vi "_PC_Daemon_Pref_SetExperimentCode.vi"(2 "error in (no error)":errorcluster, 3 "FileData":string) -> (0 "error out":errorcluster)   [LabVIEW 2018]
uses:
  RecipeEditor/Ctl/WfmCmd_Type.ctl
  PublicSubVI/Class/SigInfo/SigInfo.ctl
  PublicSubVI/Class/SigInfo/SigInfo.lvclass
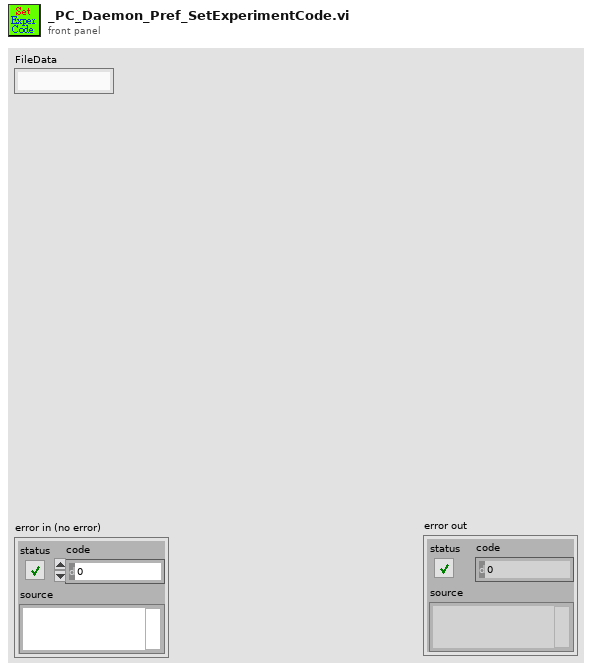
[diagram p1: front panel]
types:
  T1 = cluster{"ProcessCodes":u64[], "WfmCodes":u64[], "Signal Remarks":cluster{"mzID":u64, "SignalInfo":cluster{"Label":string, "dt":dbl, "Length":u32, "RefVolt":dbl, "mzTable":cluster{"t":dbl[], "mz":dbl[], "beta":dbl[]}}[]}, "scriptCode":string}
  T2 = typedef "SigInfo.ctl" = enum16{"New mzList", "Set SigInfo", "Get SigInfo", "Append", "End"}
  T3 = typedef "WfmCmd_Type.ctl" = enum8{"None", "WFM", "EventCodes"}
  T4 = cluster{"mzID":u64, "SignalInfo":cluster{"Label":string, "dt":dbl, "Length":u32, "RefVolt":dbl, "mzTable":cluster{"t":dbl[], "mz":dbl[], "beta":dbl[]}}[]}
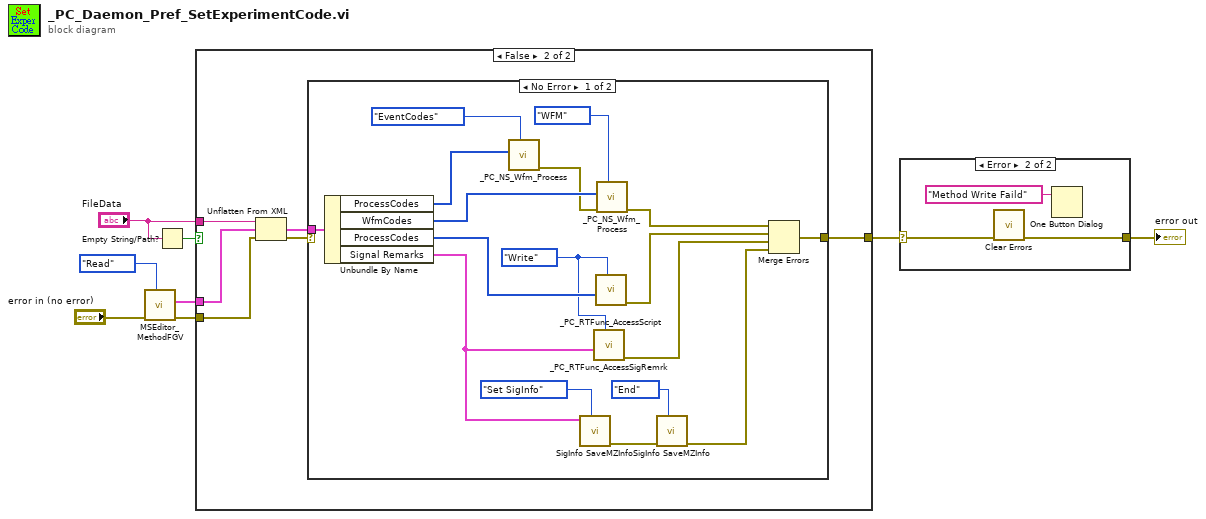
[diagram p0: block diagram]
diagram:
  n1 = call "MSEditor_MethodFGV.vi"("error in (no error)"="error in (no error)", "Function"=enum16{"Write", "Read"}."Read") -> ("Mthd out"=w4:T1, "error out"=w1:errorcluster)  [unwired: 7 in]
  n2 = Empty String/Path?(string/path="FileData") -> (empty?=w8:bool)
  n3 = case shown="False" w8 {
    tunnel: "FileData" -> [_ w14]
    tunnel: [_ w11] -> w6
    tunnel: w4 -> [_ w10]
    tunnel: w1 -> [_ w9]
    frame True {
    }
    frame False {
      n4 = Unflatten From XML(xml string=w14, type=w10, error in (no error)=w9) -> (value=w13:T1, error out=w12:errorcluster)
      n5 = case shown="No Error" w12 {
        selector: w12 -> [_ w32]
        tunnel: w13 -> [w27 _]
        tunnel: [w25 w32] -> w11
        frame No Error {
          w20 = enum16{"Write", "Read"}."Write" ("Function")
          n6 = Unbundle By Name(w27) -> ("ProcessCodes"=w29:u64[], "WfmCodes"=w28:u64[], "ProcessCodes"=w21:u64[], "Signal Remarks"=w19:T4)
          n7 = call "_PC_NS_Wfm_Process.vi"("Wfm_Type"=WfmCmd_Type."EventCodes", "WfmData_U64 in"=w29) -> ("error out"=w24:errorcluster)  [unwired: 9 in]
          n8 = call "SigInfo SaveMZInfo.vi"("Function"=SigInfo."Set SigInfo", "Signal Remarks input"=w19) -> ("error out"=w18:errorcluster)  [unwired: 7 in, 2 out]
          n9 = call "_PC_RTFunc_AccessSigRemrk.vi"("Function"=w20, "Var in"=w19) -> ("error out"=w22:errorcluster)  [unwired: 8 in, 1 out]
          n10 = call "_PC_RTFunc_AccessScript.vi"("Function"=w20, "Var in"=w21) -> ("error out"=w23:errorcluster)  [unwired: 8 in, 1 out]
          n11 = call "_PC_NS_Wfm_Process.vi"("Wfm_Type"=WfmCmd_Type."WFM", "error in (no error)"=w24, "WfmData_U64 in"=w28) -> ("error out"=w26:errorcluster)  [unwired: 8 in]
          n12 = call "SigInfo SaveMZInfo.vi"("Function"=SigInfo."End", "error in (no error)"=w18) -> ("error out"=w17:errorcluster)  [unwired: 7 in, 2 out]
          n13 = Merge Errors(w26, w23, w22, w17) -> (w25:errorcluster)
        }
        frame Error {
        }
      }
    }
  }
  n14 = case shown="Error" w6 {
    selector: w6 -> [w33 w35]
    tunnel: [w33 w34] -> w5
    frame No Error {
    }
    frame Error {
      n15 = call <vilib>:"Clear Errors.vi"("error in (no error)"=w35) -> ("error out"=w34:errorcluster)  [unwired: 5 in, 1 out]
      n16 = One Button Dialog(message="Method Write Faild") -> ()  [unwired: 1 in, 1 out]
    }
  }
  "error out" <- w5
